vi "Generate String.vi"() -> (3 "concatenated string":string)   [LabVIEW 2017]
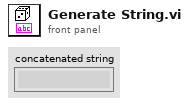
[diagram p1: front panel]
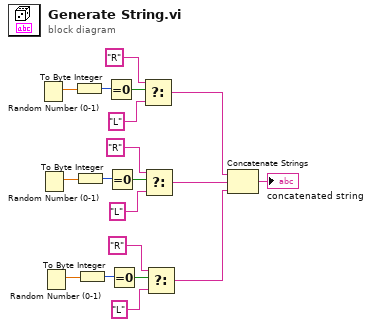
[diagram p0: block diagram]
diagram:
  n1 = Random Number (0-1)() -> (number: 0 to 1=w1:dbl)
  n2 = Random Number (0-1)() -> (number: 0 to 1=w10:dbl)
  n3 = Random Number (0-1)() -> (number: 0 to 1=w11:dbl)
  n4 = To Byte Integer(number=w1) -> (8bit integer=w2:i8)
  n5 = To Byte Integer(number=w10) -> (8bit integer=w9:i8)
  n6 = To Byte Integer(number=w11) -> (8bit integer=w12:i8)
  n7 = Equal To 0?(x=w2) -> (x = 0?=w3:bool)
  n8 = Equal To 0?(x=w9) -> (x = 0?=w8:bool)
  n9 = Equal To 0?(x=w12) -> (x = 0?=w13:bool)
  n10 = Select(t="R", s=w3, f="L") -> (s? t:f=w16:string)
  n11 = Select(t="R", s=w8, f="L") -> (s? t:f=w17:string)
  n12 = Select(t="R", s=w13, f="L") -> (s? t:f=w18:string)
  n13 = Concatenate Strings(w16, w17, w18) -> (→"concatenated string":string)
